vi "10_14_Fxp_addation.vi"(1 "y":fxp<+/-,14,10>, 2 "x":fxp<+/-,14,10>) -> (0 "x+y":fxp<+/-,15,11> format="%.41g")   [LabVIEW 2020]
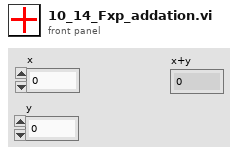
[diagram p1: front panel]
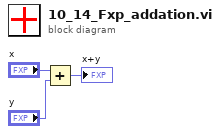
[diagram p0: block diagram]
diagram:
  n1 = Add(x="x", y="y") -> (x+y=→"x+y":fxp<+/-,15,11>)
